vi "STM.vi"() -> ()   [LabVIEW 2017, in "Konfiguracja.lvlib"]
uses:
  Libraries/Konfiguracja/Konfiguracja.lvlib
  Controls/TxA.ctl
  Controls/TxO.ctl
  Controls/Tx.ctl
  Controls/Enum_SM_read_input_write.ctl
  <vilib>/Utility/config.llb/NI_LVConfig.lvlib
panel:
  in  "Tx":T1
  in  "TxO":T2
  in  "TxA":T3
  in  "System Tab":enum32{"Termometry i paliwo"}(tab)
  in  "Etykiety T11-20":T4
  in  "Etykiety T1-10":T5
  in  "T10O":dbl
  in  "T10A":dbl
  in  "T9O":dbl
  in  "T9A":dbl
  in  "T8O":dbl
  in  "T8A":dbl
  in  "T7O":dbl
  in  "T7A":dbl
  in  "T6O":dbl
  in  "T6A":dbl
  in  "T5O":dbl
  in  "T5A":dbl
  in  "T4O":dbl
  in  "T4A":dbl
  in  "T3O":dbl
  in  "T3A":dbl
  in  "T2O":dbl
  in  "T2A":dbl
  in  "T1O":dbl
  in  "T1A":dbl
  in  "Termometr 10":bool
  in  "Termometr 9":bool
  in  "Termometr 8":bool
  in  "Termometr 7":bool
  in  "Termometr 6":bool caption="Termometr 1"
  in  "Termometr 5":bool
  in  "Termometr 4":bool
  in  "Termometr 3":bool
  in  "Termometr 2":bool
  in  "Termometr 1":bool
  in  "T20O":dbl
  in  "T20A":dbl
  in  "T19O":dbl
  in  "T19A":dbl
  in  "T18O":dbl
  in  "T18A":dbl
  in  "T17O":dbl
  in  "T17A":dbl
  in  "T16O":dbl
  in  "T16A":dbl
  in  "T15O":dbl
  in  "T15A":dbl
  in  "T14O":dbl
  in  "T14A":dbl
  in  "T13O":dbl
  in  "T13A":dbl
  in  "T12O":dbl
  in  "T12A":dbl
  in  "T11O":dbl
  in  "T11A":dbl
  in  "Termometr 20":bool
  in  "Termometr 19":bool
  in  "Termometr 18":bool
  in  "Termometr 17":bool
  in  "Termometr 16":bool caption="Termometr 1"
  in  "Termometr 15":bool
  in  "Termometr 14":bool
  in  "Termometr 13":bool
  in  "Termometr 12":bool
  in  "Termometr 11":bool caption="Termometr 1"
  in  "Czestotliwosc":dbl=0.25 min=0.25 max=60.0 step=0.25 format="%#_4g"
  in  "Port":refnum<visa-resource-name>
  in  "Copy":bool
  in  "Save":bool
  # "Zadana wartość\nostrzegawcza"
  # "Zadana wartość \nalarmowa"
  # "Zadana wartość\nostrzegawcza"
  # "Zadana wartość \nalarmowa"
  # "Etykieta"
  # "Etykieta"
  # "Częstotliwość odpytywania\n(w minutach)"
  # "Kopiuje wartośc zadaną z \npola 1 do pozostałych"
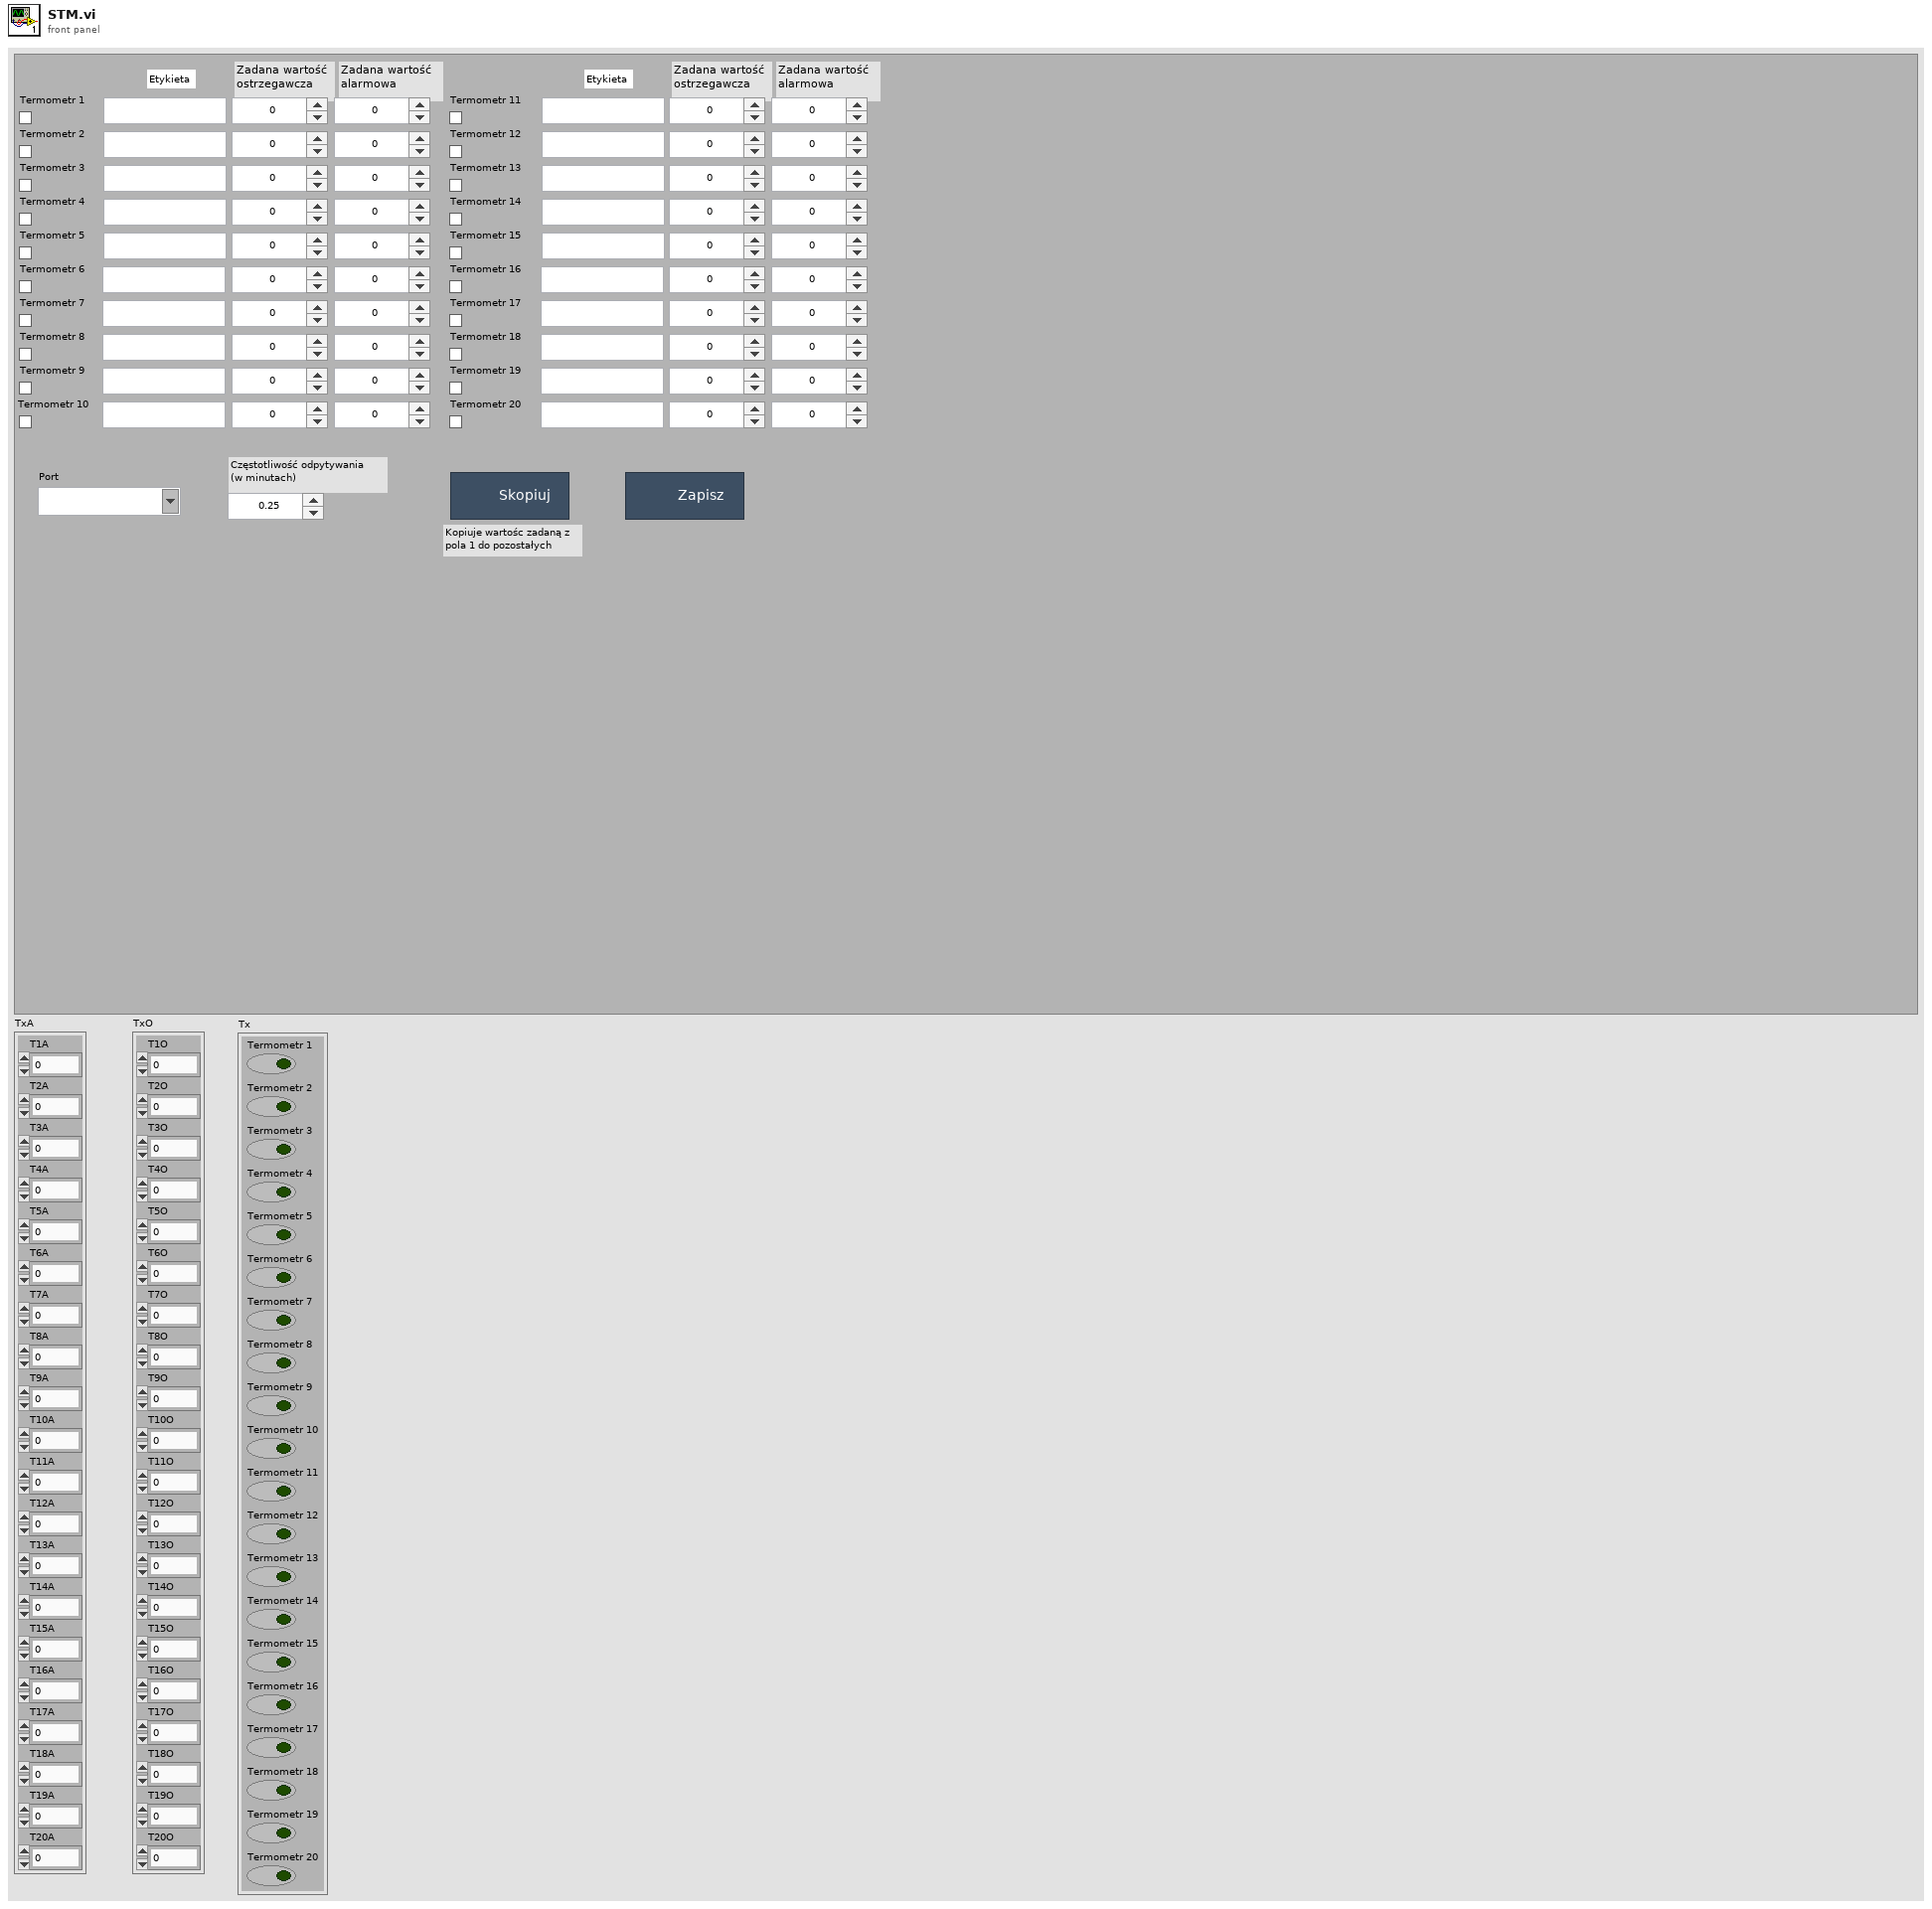
[diagram p1: front panel]
types:
  T1 = typedef "Konfiguracja.lvlib/Tx.ctl" = cluster{"Termometr 1":bool, "Termometr 2":bool, "Termometr 3":bool, "Termometr 4":bool, "Termometr 5":bool, "Termometr 6":bool, "Termometr 7":bool, "Termometr 8":bool, "Termometr 9":bool, "Termometr 10":bool, "Termometr 11":bool, "Termometr 12":bool, "Termometr 13":bool, "Termometr 14":bool, "Termometr 15":bool, "Termometr 16":bool, "Termometr 17":bool, "Termometr 18":bool, "Termometr 19":bool, "Termometr 20":bool}
  T2 = typedef "Konfiguracja.lvlib/TxO.ctl" = cluster{"T1O":dbl, "T2O":dbl, "T3O":dbl, "T4O":dbl, "T5O":dbl, "T6O":dbl, "T7O":dbl, "T8O":dbl, "T9O":dbl, "T10O":dbl, "T11O":dbl, "T12O":dbl, "T13O":dbl, "T14O":dbl, "T15O":dbl, "T16O":dbl, "T17O":dbl, "T18O":dbl, "T19O":dbl, "T20O":dbl}
  T3 = typedef "Konfiguracja.lvlib/TxA.ctl" = cluster{"T1A":dbl, "T2A":dbl, "T3A":dbl, "T4A":dbl, "T5A":dbl, "T6A":dbl, "T7A":dbl, "T8A":dbl, "T9A":dbl, "T10A":dbl, "T11A":dbl, "T12A":dbl, "T13A":dbl, "T14A":dbl, "T15A":dbl, "T16A":dbl, "T17A":dbl, "T18A":dbl, "T19A":dbl, "T20A":dbl}
  T4 = cluster{"Termometr 11":string, "Termometr 12":string, "Termometr 13":string, "Termometr 14":string, "Termometr 15":string, "Termometr 16":string, "Termometr 17":string, "Termometr 18":string, "Termometr 19":string, "Termometr 20":string}
  T5 = cluster{"Termometr 1":string, "Termometr 2":string, "Termometr 3":string, "Termometr 4":string, "Termometr 5":string, "Termometr 6":string, "Termometr 7":string, "Termometr 8":string, "Termometr 9":string, "Termometr 10":string}
  T6 = typedef "Konfiguracja.lvlib/Enum_SM_read_input_write.ctl" = enum16{"Load", "Wait for input", "Input", "Copy", "Write", "Exit"}
  T7 = typedef "NI_LVConfig.lvlib/Config Data RefNum.ctl" = refnum<k1>
  T8 = cluster{"Termometr 1":bool, "Termometr 2":bool, "Termometr 3":bool, "Termometr 4":bool, "Termometr 5":bool, "Termometr 6":bool, "Termometr 7":bool, "Termometr 8":bool, "Termometr 9":bool, "Termometr 10":bool, "Termometr 11":bool, "Termometr 12":bool, "Termometr 13":bool, "Termometr 14":bool, "Termometr 15":bool, "Termometr 16":bool, "Termometr 17":bool, "Termometr 18":bool, "Termometr 19":bool, "Termometr 20":bool}
  T9 = cluster{"T1O":dbl, "T2O":dbl, "T3O":dbl, "T4O":dbl, "T5O":dbl, "T6O":dbl, "T7O":dbl, "T8O":dbl, "T9O":dbl, "T10O":dbl, "T11O":dbl, "T12O":dbl, "T13O":dbl, "T14O":dbl, "T15O":dbl, "T16O":dbl, "T17O":dbl, "T18O":dbl, "T19O":dbl, "T20O":dbl}
  T10 = cluster{"T1A":dbl, "T2A":dbl, "T3A":dbl, "T4A":dbl, "T5A":dbl, "T6A":dbl, "T7A":dbl, "T8A":dbl, "T9A":dbl, "T10A":dbl, "T11A":dbl, "T12A":dbl, "T13A":dbl, "T14A":dbl, "T15A":dbl, "T16A":dbl, "T17A":dbl, "T18A":dbl, "T19A":dbl, "T20A":dbl}
  T11 = cluster{cluster{"T1A":dbl, "T2A":dbl, "T3A":dbl, "T4A":dbl, "T5A":dbl, "T6A":dbl, "T7A":dbl, "T8A":dbl, "T9A":dbl, "T10A":dbl, "T11A":dbl, "T12A":dbl, "T13A":dbl, "T14A":dbl, "T15A":dbl, "T16A":dbl, "T17A":dbl, "T18A":dbl, "T19A":dbl, "T20A":dbl}, cluster{"T1O":dbl, "T2O":dbl, "T3O":dbl, "T4O":dbl, "T5O":dbl, "T6O":dbl, "T7O":dbl, "T8O":dbl, "T9O":dbl, "T10O":dbl, "T11O":dbl, "T12O":dbl, "T13O":dbl, "T14O":dbl, "T15O":dbl, "T16O":dbl, "T17O":dbl, "T18O":dbl, "T19O":dbl, "T20O":dbl}, cluster{"Termometr 1":bool, "Termometr 2":bool, "Termometr 3":bool, "Termometr 4":bool, "Termometr 5":bool, "Termometr 6":bool, "Termometr 7":bool, "Termometr 8":bool, "Termometr 9":bool, "Termometr 10":bool, "Termometr 11":bool, "Termometr 12":bool, "Termometr 13":bool, "Termometr 14":bool, "Termometr 15":bool, "Termometr 16":bool, "Termometr 17":bool, "Termometr 18":bool, "Termometr 19":bool, "Termometr 20":bool}, "Port":refnum<visa-resource-name>, "Czestotliwosc":dbl, "Etykiety T1-10":cluster{"Termometr 1":string, "Termometr 2":string, "Termometr 3":string, "Termometr 4":string, "Termometr 5":string, "Termometr 6":string, "Termometr 7":string, "Termometr 8":string, "Termometr 9":string, "Termometr 10":string}, "Etykiety T11-20":cluster{"Termometr 11":string, "Termometr 12":string, "Termometr 13":string, "Termometr 14":string, "Termometr 15":string, "Termometr 16":string, "Termometr 17":string, "Termometr 18":string, "Termometr 19":string, "Termometr 20":string}}
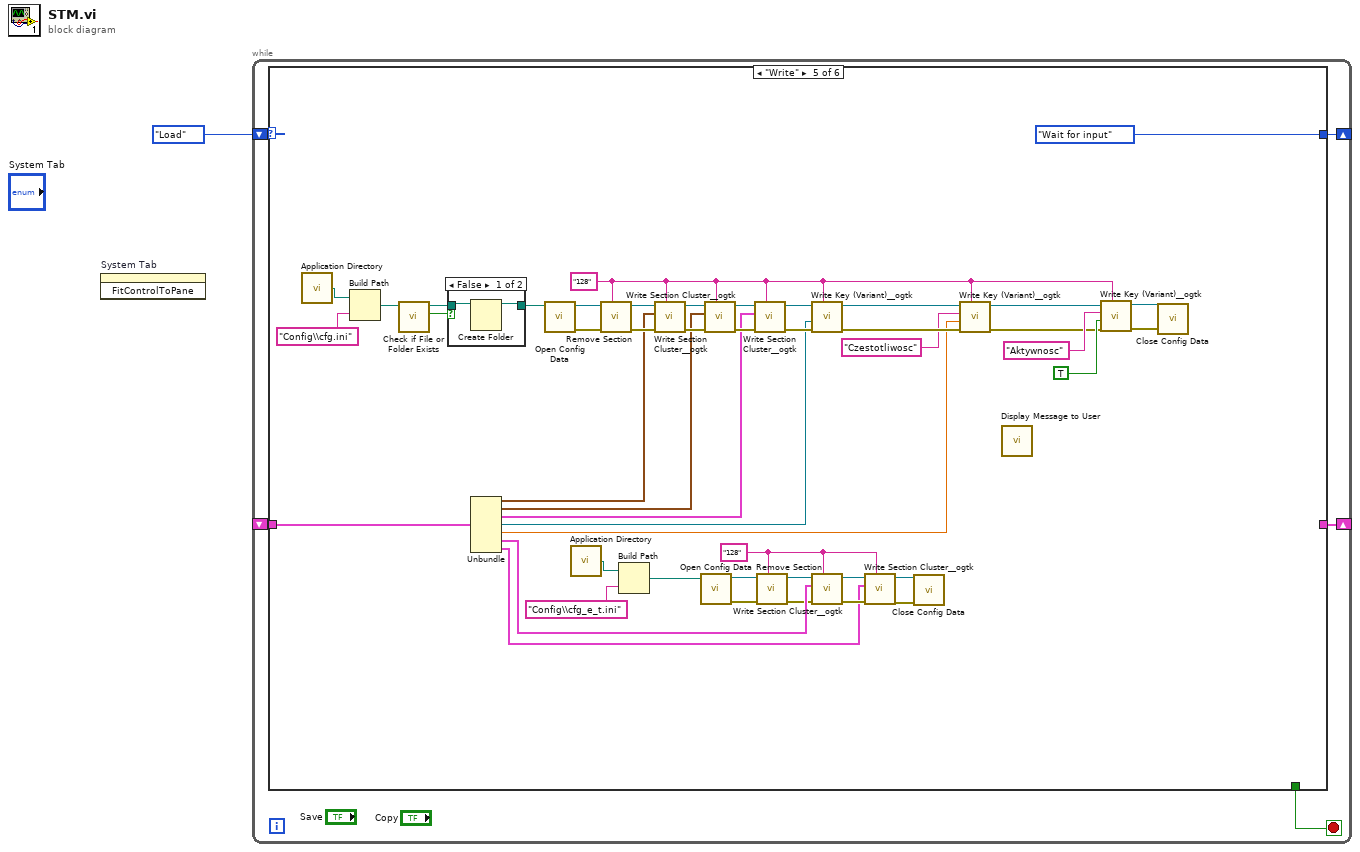
[diagram p0: block diagram]
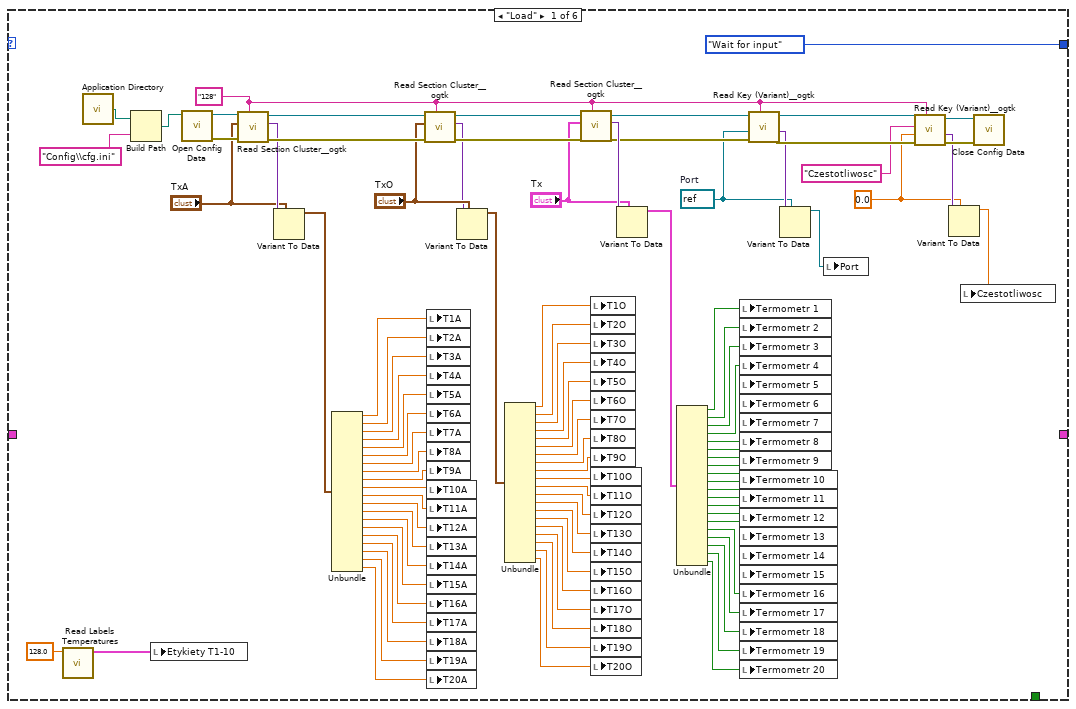
[diagram p2: hidden frame]
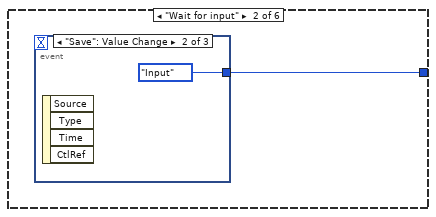
[diagram p3: hidden frame]
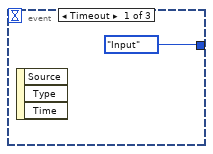
[diagram p4: hidden frame]
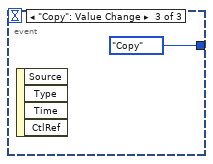
[diagram p5: hidden frame]
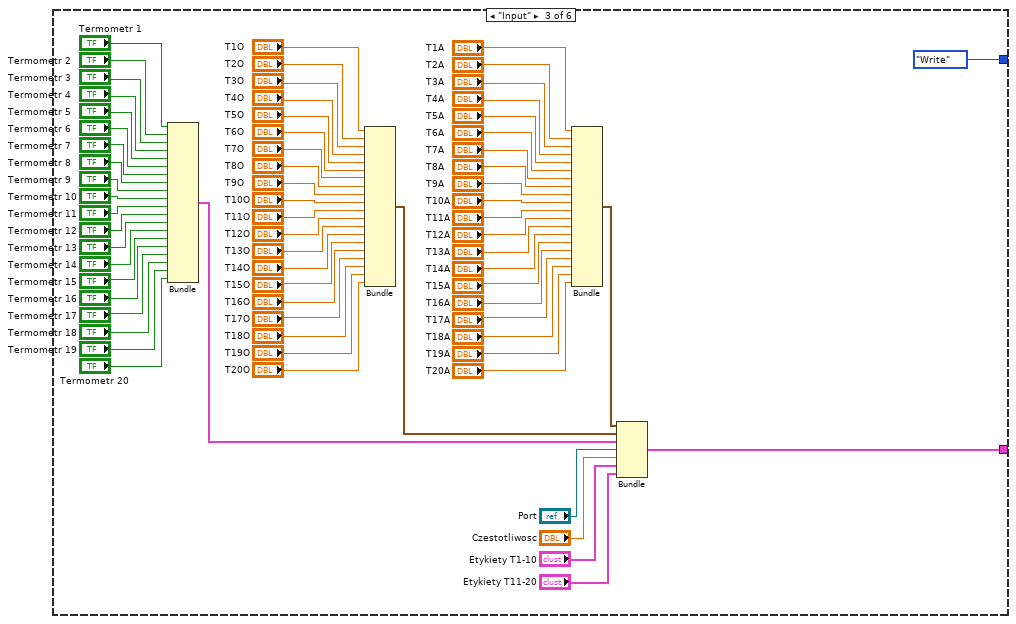
[diagram p6: hidden frame]
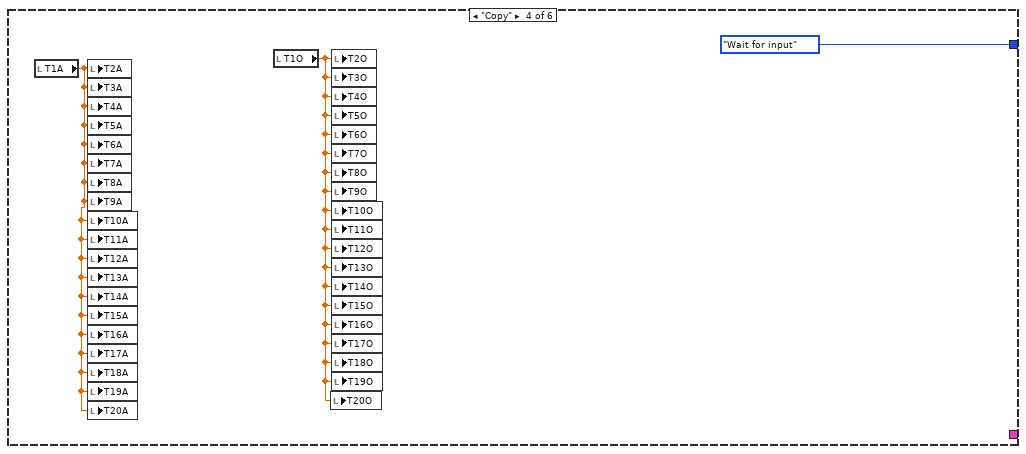
[diagram p7: hidden frame]
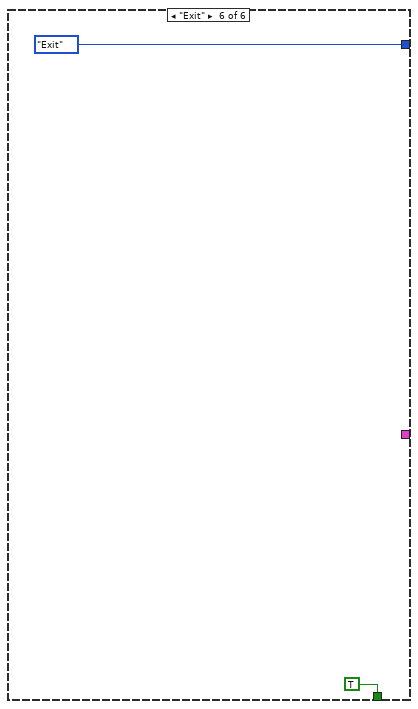
[diagram p9: hidden frame]
diagram:
  n1 = invoke on="System Tab" class="TabCtl (strict)" method="FitControlToPane"() -> ()  [unwired: 3 in, 3 out]
  n2 = while {
    shift-right: [w5] -> _
    shift-left: Enum_SM_read_input_write."Load" -> [w6]
    shift-right: [w4] -> _
    shift-left: _ -> [w3]
    stop <- w2 stop-if-true
    n3 = case shown="\"Write\"" w6 {
      tunnel: [Enum_SM_read_input_write."Wait for input" w102 Enum_SM_read_input_write."Write" Enum_SM_read_input_write."Wait for input" Enum_SM_read_input_write."Wait for input" Enum_SM_read_input_write."Exit"] -> w5
      tunnel: [_ _ w111 _ _ _] -> w4
      tunnel: w3 -> [_ _ _ _ w221 _]
      tunnel: [_ _ _ _ _ TRUE] -> w2
      frame "Load" {
        w9 = 0.0
        w18 = refnum<visa-resource-name> refnum  # Port
        w13 = "128" ("section (optional)")
        n4 = call "Read Labels Temperatures.vi"("Slave ID"=128.0) -> ("Etykiety T1-10"=w8:T5)  [unwired: 10 in]
        n5 = call <vilib>:"Application Directory.vi"() -> ("Application Directory"=w99:path)
        n6 = Build Path(base path=w99, name or relative path="Config\\cfg.ini") -> (appended path=w97:path)
        n7 = local write "Etykiety T1-10"(w8) -> ()
        n8 = call <vilib>:"Open Config Data.vi"("configuration file path"=w97) -> ("error out"=w96:errorcluster, "refnum"=w95:T7)  [unwired: 8 in, 1 out]
        n9 = call <userlib>:"Read Section Cluster__ogtk.vi"("section (optional)"=w13, "error in (no error)"=w96, "Section Formatted Cluster Type"="TxA", "refnum"=w95) -> ("error out"=w94:errorcluster, "Section Formatted Cluster"=w90:variant, "dup refnum"=w93:T7)  [unwired: 3 in, 2 out]
        n10 = Variant To Data(type="TxA", Variant=w90) -> (data=w88:T3)  [unwired: 1 in, 1 out]
        n11 = Unbundle(w88) -> ("T1A"=w68:dbl, "T2A"=w69:dbl, "T3A"=w70:dbl, "T4A"=w71:dbl, "T5A"=w72:dbl, "T6A"=w73:dbl, "T7A"=w74:dbl, "T8A"=w75:dbl, "T9A"=w76:dbl, "T10A"=w77:dbl, "T11A"=w78:dbl, "T12A"=w79:dbl, "T13A"=w80:dbl, "T14A"=w81:dbl, "T15A"=w82:dbl, "T16A"=w83:dbl, "T17A"=w84:dbl, "T18A"=w85:dbl, "T19A"=w86:dbl, "T20A"=w87:dbl)
        n12 = call <userlib>:"Read Section Cluster__ogtk.vi"("section (optional)"=w13, "error in (no error)"=w94, "Section Formatted Cluster Type"="TxO", "refnum"=w93) -> ("error out"=w92:errorcluster, "Section Formatted Cluster"=w45:variant, "dup refnum"=w91:T7)  [unwired: 3 in, 2 out]
        n13 = local write "T1A"(w68) -> ()
        n14 = local write "T2A"(w69) -> ()
        n15 = local write "T3A"(w70) -> ()
        n16 = local write "T4A"(w71) -> ()
        n17 = local write "T5A"(w72) -> ()
        n18 = local write "T6A"(w73) -> ()
        n19 = local write "T7A"(w74) -> ()
        n20 = local write "T8A"(w75) -> ()
        n21 = local write "T9A"(w76) -> ()
        n22 = local write "T10A"(w77) -> ()
        n23 = local write "T11A"(w78) -> ()
        n24 = local write "T12A"(w79) -> ()
        n25 = local write "T13A"(w80) -> ()
        n26 = local write "T14A"(w81) -> ()
        n27 = local write "T15A"(w82) -> ()
        n28 = local write "T16A"(w83) -> ()
        n29 = local write "T17A"(w84) -> ()
        n30 = local write "T18A"(w85) -> ()
        n31 = local write "T19A"(w86) -> ()
        n32 = local write "T20A"(w87) -> ()
        n33 = Variant To Data(type="TxO", Variant=w45) -> (data=w67:T2)  [unwired: 1 in, 1 out]
        n34 = Unbundle(w67) -> ("T1O"=w47:dbl, "T2O"=w48:dbl, "T3O"=w49:dbl, "T4O"=w50:dbl, "T5O"=w51:dbl, "T6O"=w52:dbl, "T7O"=w53:dbl, "T8O"=w54:dbl, "T9O"=w55:dbl, "T10O"=w56:dbl, "T11O"=w57:dbl, "T12O"=w58:dbl, "T13O"=w59:dbl, "T14O"=w60:dbl, "T15O"=w61:dbl, "T16O"=w62:dbl, "T17O"=w63:dbl, "T18O"=w64:dbl, "T19O"=w65:dbl, "T20O"=w66:dbl)
        n35 = call <userlib>:"Read Section Cluster__ogtk.vi"("section (optional)"=w13, "error in (no error)"=w92, "Section Formatted Cluster Type"="Tx", "refnum"=w91) -> ("error out"=w20:errorcluster, "Section Formatted Cluster"=w44:variant, "dup refnum"=w21:T7)  [unwired: 3 in, 2 out]
        n36 = local write "T1O"(w47) -> ()
        n37 = local write "T2O"(w48) -> ()
        n38 = local write "T3O"(w49) -> ()
        n39 = local write "T4O"(w50) -> ()
        n40 = local write "T5O"(w51) -> ()
        n41 = local write "T6O"(w52) -> ()
        n42 = local write "T7O"(w53) -> ()
        n43 = local write "T8O"(w54) -> ()
        n44 = local write "T9O"(w55) -> ()
        n45 = local write "T10O"(w56) -> ()
        n46 = local write "T11O"(w57) -> ()
        n47 = local write "T12O"(w58) -> ()
        n48 = local write "T13O"(w59) -> ()
        n49 = local write "T14O"(w60) -> ()
        n50 = local write "T15O"(w61) -> ()
        n51 = local write "T16O"(w62) -> ()
        n52 = local write "T17O"(w63) -> ()
        n53 = local write "T18O"(w64) -> ()
        n54 = local write "T19O"(w65) -> ()
        n55 = local write "T20O"(w66) -> ()
        n56 = Variant To Data(type="Tx", Variant=w44) -> (data=w22:T1)  [unwired: 1 in, 1 out]
        n57 = Unbundle(w22) -> ("Termometr 1"=w23:bool, "Termometr 2"=w24:bool, "Termometr 3"=w25:bool, "Termometr 4"=w26:bool, "Termometr 5"=w27:bool, "Termometr 6"=w28:bool, "Termometr 7"=w29:bool, "Termometr 8"=w30:bool, "Termometr 9"=w31:bool, "Termometr 10"=w32:bool, "Termometr 11"=w33:bool, "Termometr 12"=w34:bool, "Termometr 13"=w35:bool, "Termometr 14"=w36:bool, "Termometr 15"=w37:bool, "Termometr 16"=w38:bool, "Termometr 17"=w39:bool, "Termometr 18"=w40:bool, "Termometr 19"=w41:bool, "Termometr 20"=w42:bool)
        n58 = local write "Termometr 1"(w23) -> ()
        n59 = local write "Termometr 2"(w24) -> ()
        n60 = local write "Termometr 3"(w25) -> ()
        n61 = local write "Termometr 4"(w26) -> ()
        n62 = local write "Termometr 5"(w27) -> ()
        n63 = local write "Termometr 6"(w28) -> ()
        n64 = local write "Termometr 7"(w29) -> ()
        n65 = local write "Termometr 8"(w30) -> ()
        n66 = local write "Termometr 9"(w31) -> ()
        n67 = local write "Termometr 10"(w32) -> ()
        n68 = local write "Termometr 11"(w33) -> ()
        n69 = local write "Termometr 12"(w34) -> ()
        n70 = local write "Termometr 13"(w35) -> ()
        n71 = local write "Termometr 14"(w36) -> ()
        n72 = local write "Termometr 15"(w37) -> ()
        n73 = local write "Termometr 16"(w38) -> ()
        n74 = local write "Termometr 17"(w39) -> ()
        n75 = local write "Termometr 18"(w40) -> ()
        n76 = local write "Termometr 19"(w41) -> ()
        n77 = local write "Termometr 20"(w42) -> ()
        n78 = call <userlib>:"Read Key (Variant)__ogtk.vi"("section"=w13, "error in (no error)"=w20, "type"=w18, "refnum"=w21) -> ("error out"=w101:errorcluster, "key-value"=w19:variant, "refnum out"=w16:T7)  [unwired: 4 in, 1 out]
        n79 = Variant To Data(type=w18, Variant=w19) -> (data=w17:refnum<visa-resource-name>)  [unwired: 1 in, 1 out]
        n80 = local write "Port"(w17) -> ()
        n81 = call <userlib>:"Read Key (Variant)__ogtk.vi"("section"=w13, "error in (no error)"=w101, "type"=w9, "key (optional)"="Czestotliwosc", "refnum"=w16) -> ("error out"=w14:errorcluster, "key-value"=w11:variant, "refnum out"=w15:T7)  [unwired: 3 in, 1 out]
        n82 = Variant To Data(type=w9, Variant=w11) -> (data=w10:dbl)  [unwired: 1 in, 1 out]
        n83 = local write "Czestotliwosc"(w10) -> ()
        n84 = call <vilib>:"Close Config Data.vi"("error in (no error)"=w14, "refnum"=w15) -> ()  [unwired: 8 in, 2 out]
      }
      frame "Wait for input" {
        n85 = event shown="[1] \"Save\": Value Change" {
          selector: _ -> [_ _ _]
          dyn-events: _ -> [_ _ _]
          timeout: _ -> [_ _ _]
          tunnel: [Enum_SM_read_input_write."Input" Enum_SM_read_input_write."Input" Enum_SM_read_input_write."Copy"] -> w102
          event Timeout {
            n86 = event-data() -> ()  [unwired: 1 in, 3 out]
          }
          event "Save": Value Change {
            n87 = event-data() -> ()  [unwired: 1 in, 4 out]
          }
          event "Copy": Value Change {
            n88 = event-data() -> ()  [unwired: 1 in, 4 out]
          }
        }
      }
      frame "Input" {
        n89 = Bundle("Termometr 1"="Termometr 1", "Termometr 2"="Termometr 2", "Termometr 3"="Termometr 3", "Termometr 4"="Termometr 4", "Termometr 5"="Termometr 5", "Termometr 6"="Termometr 6", "Termometr 7"="Termometr 7", "Termometr 8"="Termometr 8", "Termometr 9"="Termometr 9", "Termometr 10"="Termometr 10", "Termometr 11"="Termometr 11", "Termometr 12"="Termometr 12", "Termometr 13"="Termometr 13", "Termometr 14"="Termometr 14", "Termometr 15"="Termometr 15", "Termometr 16"="Termometr 16", "Termometr 17"="Termometr 17", "Termometr 18"="Termometr 18", "Termometr 19"="Termometr 19", "Termometr 20"="Termometr 20") -> (w112:T8)  [unwired: 1 in]
        n90 = Bundle("T1O"="T1O", "T2O"="T2O", "T3O"="T3O", "T4O"="T4O", "T5O"="T5O", "T6O"="T6O", "T7O"="T7O", "T8O"="T8O", "T9O"="T9O", "T10O"="T10O", "T11O"="T11O", "T12O"="T12O", "T13O"="T13O", "T14O"="T14O", "T15O"="T15O", "T16O"="T16O", "T17O"="T17O", "T18O"="T18O", "T19O"="T19O", "T20O"="T20O") -> (w113:T9)  [unwired: 1 in]
        n91 = Bundle("T1A"="T1A", "T2A"="T2A", "T3A"="T3A", "T4A"="T4A", "T5A"="T5A", "T6A"="T6A", "T7A"="T7A", "T8A"="T8A", "T9A"="T9A", "T10A"="T10A", "T11A"="T11A", "T12A"="T12A", "T13A"="T13A", "T14A"="T14A", "T15A"="T15A", "T16A"="T16A", "T17A"="T17A", "T18A"="T18A", "T19A"="T19A", "T20A"="T20A") -> (w114:T10)  [unwired: 1 in]
        n92 = Bundle(w114, w113, w112, "Port"="Port", "Czestotliwosc"="Czestotliwosc", "Etykiety T1-10"="Etykiety T1-10", "Etykiety T11-20"="Etykiety T11-20") -> (w111:T11)  [unwired: 1 in]
      }
      frame "Copy" {
        n93 = local read "T1A"() -> (w176:dbl)
        n94 = local write "T2A"(w176) -> ()
        n95 = local write "T3A"(w176) -> ()
        n96 = local write "T4A"(w176) -> ()
        n97 = local write "T5A"(w176) -> ()
        n98 = local write "T6A"(w176) -> ()
        n99 = local write "T7A"(w176) -> ()
        n100 = local write "T8A"(w176) -> ()
        n101 = local write "T9A"(w176) -> ()
        n102 = local write "T10A"(w176) -> ()
        n103 = local write "T11A"(w176) -> ()
        n104 = local write "T12A"(w176) -> ()
        n105 = local write "T13A"(w176) -> ()
        n106 = local write "T14A"(w176) -> ()
        n107 = local write "T15A"(w176) -> ()
        n108 = local write "T16A"(w176) -> ()
        n109 = local write "T17A"(w176) -> ()
        n110 = local write "T18A"(w176) -> ()
        n111 = local write "T19A"(w176) -> ()
        n112 = local write "T20A"(w176) -> ()
        n113 = local read "T1O"() -> (w175:dbl)
        n114 = local write "T20O"(w175) -> ()
        n115 = local write "T2O"(w175) -> ()
        n116 = local write "T3O"(w175) -> ()
        n117 = local write "T4O"(w175) -> ()
        n118 = local write "T5O"(w175) -> ()
        n119 = local write "T6O"(w175) -> ()
        n120 = local write "T7O"(w175) -> ()
        n121 = local write "T8O"(w175) -> ()
        n122 = local write "T9O"(w175) -> ()
        n123 = local write "T10O"(w175) -> ()
        n124 = local write "T11O"(w175) -> ()
        n125 = local write "T12O"(w175) -> ()
        n126 = local write "T13O"(w175) -> ()
        n127 = local write "T14O"(w175) -> ()
        n128 = local write "T15O"(w175) -> ()
        n129 = local write "T16O"(w175) -> ()
        n130 = local write "T17O"(w175) -> ()
        n131 = local write "T18O"(w175) -> ()
        n132 = local write "T19O"(w175) -> ()
      }
      frame "Write" {
        w185 = "128" ("section")
        w202 = "128" ("section (optional)")
        n133 = call <vilib>:"Application Directory.vi"() -> ("Application Directory"=w223:path)
        n134 = Build Path(base path=w223, name or relative path="Config\\cfg.ini") -> (appended path=w181:path)
        n135 = call <vilib>:"Check if File or Folder Exists.vi"("path"=w181) -> ("file or folder exists?"=w180:bool, "dup path"=w179:path)  [unwired: 8 in, 1 out]
        n136 = case shown="False" w180 {
          tunnel: w179 -> [w226 w227]
          tunnel: [w225 w227] -> w178
          frame False {
            n137 = Create Folder(path (use dialog)=w226) -> (created path=w225:path)  [unwired: 2 in, 2 out]
          }
          frame True {
          }
        }
        n138 = Unbundle(w221) -> (w212:T10, w211:T9, w210:T8, "Port"=w207:refnum<visa-resource-name>, "Czestotliwosc"=w199:dbl, "Etykiety T1-10"=w189:T5, "Etykiety T11-20"=w184:T4)
        n139 = call <vilib>:"Open Config Data.vi"("configuration file path"=w178) -> ("error out"=w213:errorcluster, "refnum"=w216:T7)  [unwired: 8 in, 1 out]
        n140 = call <vilib>:"Application Directory.vi"() -> ("Application Directory"=w191:path)
        n141 = call <vilib>:"Remove Section.vi"("section"=w202, "error in (no error)"=w213, "refnum"=w216) -> ("error out"=w214:errorcluster, "refnum out"=w215:T7)  [unwired: 6 in, 1 out]
        n142 = Build Path(base path=w191, name or relative path="Config\\cfg_e_t.ini") -> (appended path=w194:path)
        n143 = call <userlib>:"Write Section Cluster__ogtk.vi"("section (optional)"=w202, "error in (no error)"=w214, "Section Formatted Cluster"=w212, "refnum"=w215) -> ("error out"=w218:errorcluster, "dup refnum"=w220:T7)  [unwired: 6 in]
        n144 = call <vilib>:"Open Config Data.vi"("configuration file path"=w194) -> ("error out"=w192:errorcluster, "refnum"=w193:T7)  [unwired: 8 in, 1 out]
        n145 = call <userlib>:"Write Section Cluster__ogtk.vi"("section (optional)"=w202, "error in (no error)"=w218, "Section Formatted Cluster"=w211, "refnum"=w220) -> ("error out"=w217:errorcluster, "dup refnum"=w219:T7)  [unwired: 6 in]
        n146 = call <userlib>:"Write Section Cluster__ogtk.vi"("section (optional)"=w202, "error in (no error)"=w217, "Section Formatted Cluster"=w210, "refnum"=w219) -> ("error out"=w209:errorcluster, "dup refnum"=w208:T7)  [unwired: 6 in]
        n147 = call <vilib>:"Remove Section.vi"("section"=w185, "error in (no error)"=w192, "refnum"=w193) -> ("error out"=w188:errorcluster, "refnum out"=w190:T7)  [unwired: 6 in, 1 out]
        n148 = call <userlib>:"Write Key (Variant)__ogtk.vi"("section"=w202, "error in (no error)"=w209, "key-value"=w207, "refnum"=w208) -> ("error out"=w200:errorcluster, "refnum out"=w201:T7)  [unwired: 6 in]
        n149 = call <userlib>:"Write Section Cluster__ogtk.vi"("section (optional)"=w185, "error in (no error)"=w188, "Section Formatted Cluster"=w189, "refnum"=w190) -> ("error out"=w187:errorcluster, "dup refnum"=w186:T7)  [unwired: 6 in]
        n150 = call <userlib>:"Write Section Cluster__ogtk.vi"("section (optional)"=w185, "error in (no error)"=w187, "Section Formatted Cluster"=w184, "refnum"=w186) -> ("error out"=w182:errorcluster, "dup refnum"=w183:T7)  [unwired: 6 in]
        n151 = call <vilib>:"Close Config Data.vi"("error in (no error)"=w182, "refnum"=w183) -> ()  [unwired: 8 in, 2 out]
        n152 = call <userlib>:"Write Key (Variant)__ogtk.vi"("section"=w202, "error in (no error)"=w200, "key-value"=w199, "key (optional)"="Czestotliwosc", "refnum"=w201) -> ("error out"=w198:errorcluster, "refnum out"=w197:T7)  [unwired: 5 in]
        n153 = call "Display Message to User"() -> ()  [unwired: 10 in, 2 out]
        n154 = call <userlib>:"Write Key (Variant)__ogtk.vi"("section"=w202, "error in (no error)"=w198, "key-value"=TRUE, "key (optional)"="Aktywnosc", "refnum"=w197) -> ("error out"=w205:errorcluster, "refnum out"=w206:T7)  [unwired: 5 in]
        n155 = call <vilib>:"Close Config Data.vi"("error in (no error)"=w205, "refnum"=w206) -> ()  [unwired: 8 in, 2 out]
      }
      frame "Exit" {
      }
    }
  }
